vi "get pthread error.vi"(7 "function":T1=enum."pthread_cond_broadcast", 8 "error in (no error)":errorcluster, 11 "errno":i32) -> (0 "error out":errorcluster)   [LabVIEW 2013, in "Linux RT IPC.POSIX Threads.lvlib" / "POSIX Thread Object.lvclass"]
uses:
  <vilib>/NI/NI Linux RT IPC/POSIX Threads/Classes/POSIX Thread Object/POSIX Thread Object.lvclass
  <vilib>/NI/NI Linux RT Errno/Linux Errno.lvlib
  <vilib>/NI/NI Linux RT IPC/POSIX Threads/Classes/POSIX Thread Object/Controls/pthread functions.ctl
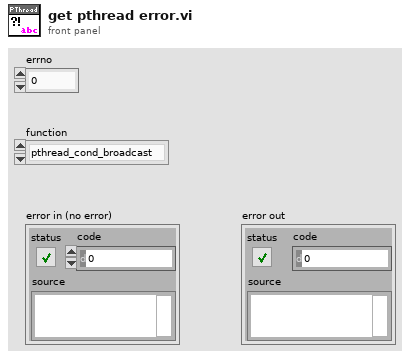
[diagram p1: front panel]
types:
  T1 = typedef "Linux RT IPC.POSIX Threads.lvlib/POSIX Thread Object.lvclass/pthread functions.ctl" = enum16{"unspecified", "pthread_condattr_init", "pthread_condattr_destroy", "pthread_condattr_getclock", "pthread_condattr_setclock", "pthread_condattr_getpshared", "pthread_condattr_setpshared", "pthread_cond_init", "pthread_cond_destroy", "pthread_cond_broadcast", "pthread_cond_signal", "pthread_cond_timedwait", "pthread_cond_wait", "pthread_mutexattr_init", "pthread_mutexattr_destroy", "pthread_mutexattr_getprioceiling", "pthread_mutexattr_setprioceiling", "pthread_mutexattr_getprotocol", "pthread_mutexattr_setprotocol", "pthread_mutexattr_getpshared", "pthread_mutexattr_setpshared", "pthread_mutexattr_gettype", "pthread_mutexattr_settype", "pthread_mutex_init", "pthread_mutex_destroy", "pthread_mutex_getprioceiling", "pthread_mutex_setprioceiling", "pthread_mutex_lock", "pthread_mutex_timedlock", "pthread_mutex_trylock", "pthread_mutex_unlock", "sem_destroy", "sem_getvalue", "sem_init", "sem_open", "sem_post", "sem_timedwait", "sem_trywait", "sem_wait", "barrier_init", "barrier_destroy", "barrier_wait", "barrierattr_init", "barrierattr_destroy", "barrierattr_getpshared", "barrierattr_setpshared"}
  T2 = typedef "Linux Errno.lvlib/errno.ctl" = enum16{"NO ERROR", "EPERM", "ENOENT", "ESRCH", "EINTR", "EIO", "ENXIO", "E2BIG", "ENOEXEC", "EBADF", "ECHILD", "EAGAIN", "ENOMEM", "EACCES", "EFAULT", "ENOTBLK", "EBUSY", "EEXIST", "EXDEV", "ENODEV", "ENOTDIR", "EISDIR", "EINVAL", "ENFILE", "EMFILE", "ENOTTY", "ETXTBSY", "EFBIG", "ENOSPC", "ESPIPE", "EROFS", "EMLINK", "EPIPE", "EDOM", "ERANGE", "EDADLK", "ENAMETOOLONG", "ENOLCK", "ENOSYS", "ENOTEMPTY", "ELOOP", "EWOULDBLOCK", "ENOMSG", "EIDRM", "ECHRNG", "EL2NSYNC", "EL3HLT", "EL3RST", "ELNRNG", "EUNATCH", "ENOCSI", "EL2HLT", "EBADE", "EBADR", "EXFULL", "ENOANO", "EBADRQC", "EBADSLT", "EDEADLOCK", "EBFONT", "ENOSTR", "ENODATA", "ETIME", "ENOSR", "ENONET", "ENOPKG", "EREMOTE", "ENOLINK", "EADV", "ESRMNT", "ECOMM", "EPROTO", "EMULTIHOP", "EDOTDOT", "EBADMSG", "EOVERFLOW", "ENOTUNIQ", "EBADFD", "EREMCHG", "ELIBACC", "ELIBBAD", "ELIBSCN", "ELIBMAX", "ELIBEXEC", "ELISEQ", "ERESTART", "ESTRPIPE", "EUSERS", "ENOTSOCK", "EDESTADDRREQ", "EMSGSIZE", "EPROTOTYPE", "ENOPROTOOPT", "EPROTONOSUPPORT", "ESOCKTNOSUPPORT", "EOPNOTSUPP", "EPFNOSUPPORT", "EAFNOSUPPORT", "EADDRINUSE", "EADDRNOTAVAIL", "ENETDOWN", "ENETUNREACH", "ENETRESET", "ECONNABORTED", "ECONNRESET", "ENOBUFS", "EISCONN", "ENOTCONN", "ESHUTDOWN", "ETOOMANYREFS", "ETIMEDOUT", "ECONNREFUSED", "EHOSTDOWN", "EHOSTUNREACH", "EALREADY", "EINPROGRESS", "ESTALE", "EUCLEAN", "ENOTNAM", "ENAVAIL", "EISNAM", "EREMOTEIO", "EDQUOT", "ENOMEDIUM", "EMEDIUMTYPE", "ECANCELED", "ENOKEY", "EKEYEXPIRED", "EKEYREVOKED", "EKEYREJECTED", "EOWNERDEAD", "ENOTRECOVERABLE", "ERFKILL", "EHWPOISON", "UNDEFINED"}
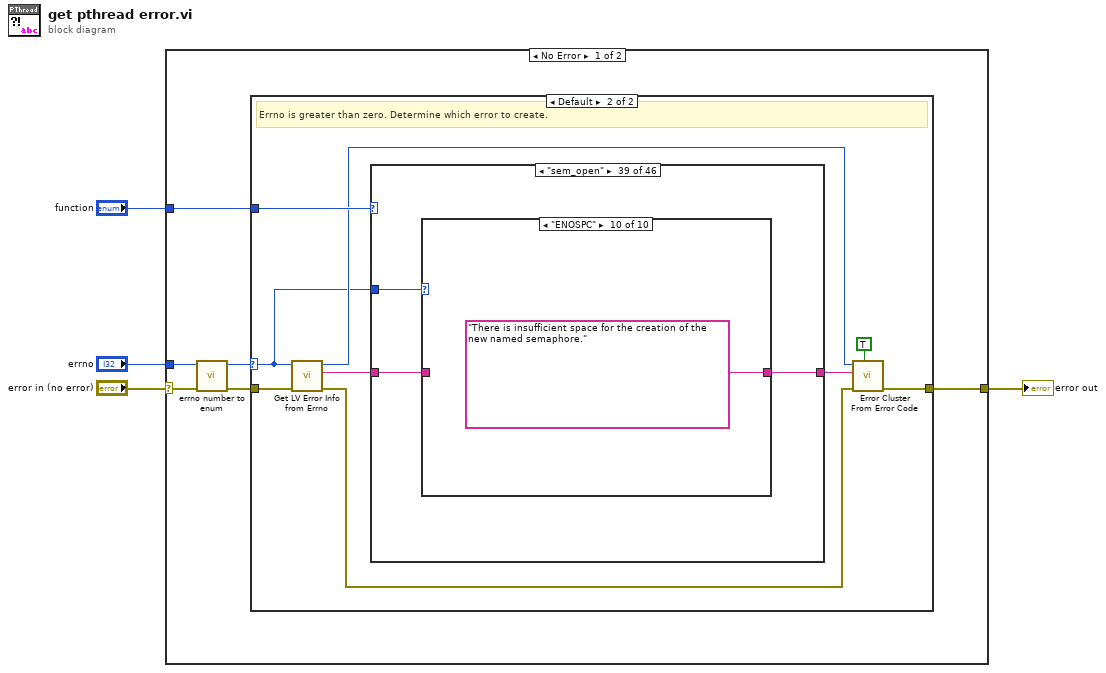
[diagram p0: block diagram]
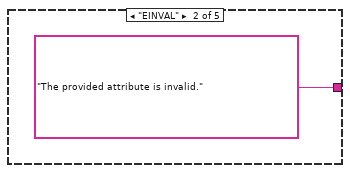
[diagram p5: hidden frame]
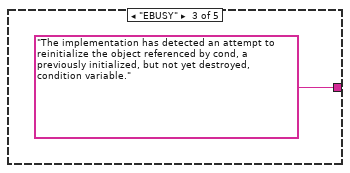
[diagram p6: hidden frame]
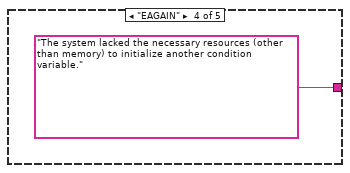
[diagram p7: hidden frame]
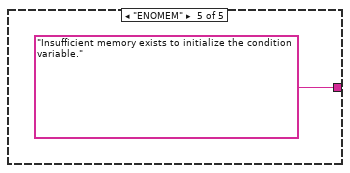
[diagram p8: hidden frame]
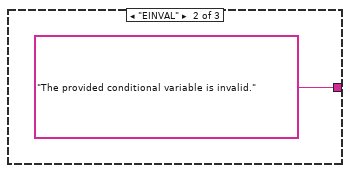
[diagram p10: hidden frame]
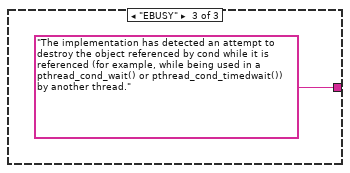
[diagram p11: hidden frame]
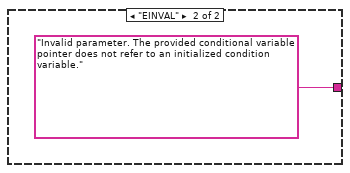
[diagram p13: hidden frame]
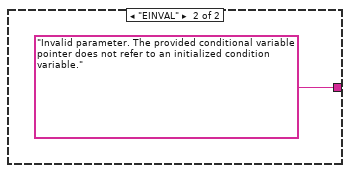
[diagram p15: hidden frame]
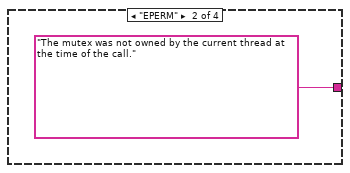
[diagram p17: hidden frame]
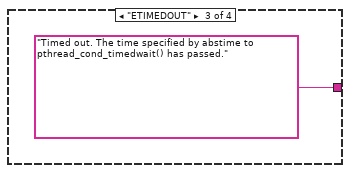
[diagram p18: hidden frame]
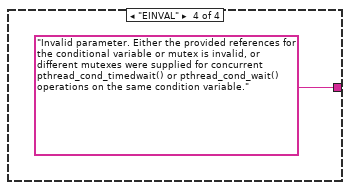
[diagram p19: hidden frame]
diagram:
  n1 = case shown="No Error" "error in (no error)" {
    selector: "error in (no error)" -> [w8 w295]
    tunnel: [w10 w295] -> w3
    tunnel: "errno" -> [w7 _]
    tunnel: "function" -> [w9 _]
    frame No Error {
      n2 = call <vilib>:"errno number to enum.vi"("error in (no error)"=w8, "errno number"=w7) -> ("error out"=w6:errorcluster, "errno enum"=w5:T2)  [unwired: 8 in]
      n3 = case shown="Default" w5 {
        selector: w5 -> [_ w12]
        tunnel: [w11 w20] -> w10
        tunnel: w9 -> [_ w19]
        tunnel: w6 -> [w11 w13]
        frame "NO ERROR" {
          # "Errno is zero. No error occurred."
        }
        frame Default {
          # "Errno is greater than zero. Determine which error to create."
          n4 = call <vilib>:"Get LV Error Info from Errno.vi"("error in (no error)"=w13, "errno"=w12) -> ("error out"=w15:errorcluster, "error description"=w16:string, "error code"=w14:i32)  [unwired: 7 in]
          n5 = case shown="\"sem_open\"" w19 {
            tunnel: w12 -> [_ w24 w32 w38 w43 w48 w55 w61 w66 w71 w76 w81 w86 w91 w96 w101 w107 w113 w119 w126 w131 w136 w141 w146 w155 w161 w167 w173 w181 w189 w196 w203 w208 w213 w219 w225 w232 w239 w245 w258 w266 w272 w277 w282 w287 w292]
            tunnel: [w21 w23 w31 w37 w42 w47 w54 w60 w65 w70 w75 w80 w85 w90 w95 w100 w106 w112 w118 w125 w130 w135 w140 w145 w154 w160 w166 w172 w180 w188 w195 w202 w207 w212 w218 w224 w231 w238 w244 w257 w265 w271 w276 w281 w286 w291] -> w17
            tunnel: w16 -> [w21 w22 w30 w36 w41 w46 w53 w59 w64 w69 w74 w79 w84 w89 w94 w99 w105 w111 w117 w124 w129 w134 w139 w144 w153 w159 w165 w171 w179 w187 w194 w201 w206 w211 w217 w223 w230 w237 w243 w256 w264 w270 w275 w280 w285 w290]
            frame "unspecified", Default {
              # "No specific function was specified, so use generic error description."
            }
            frame "pthread_cond_init" {
              n6 = case shown="\"NO ERROR\", Default" w24 {
                tunnel: [w25 "The provided attribute is invalid." "The implementation has detected an attempt to reinitialize the object referenced by cond, a previously initialized, but not yet destroyed, condition variable." "The system lacked the necessary resources (other than memory) to initialize another condition variable." "Insufficient memory exists to initialize the condition variable."] -> w23
                tunnel: w22 -> [w25 _ _ _ _]
                frame "NO ERROR", Default {
                }
                frame "EINVAL" {
                }
                frame "EBUSY" {
                }
                frame "EAGAIN" {
                }
                frame "ENOMEM" {
                }
              }
            }
            frame "pthread_cond_destroy" {
              n7 = case shown="\"NO ERROR\", Default" w32 {
                tunnel: [w33 "The provided conditional variable is invalid." "The implementation has detected an attempt to destroy the object referenced by cond while it is referenced (for example, while being used in a pthread_cond_wait() or pthread_cond_timedwait()) by another thread."] -> w31
                tunnel: w30 -> [w33 _ _]
                frame "NO ERROR", Default {
                }
                frame "EINVAL" {
                }
                frame "EBUSY" {
                }
              }
            }
            frame "pthread_cond_broadcast" {
              n8 = case shown="\"NO ERROR\", Default" w38 {
                tunnel: [w39 "Invalid parameter. The provided conditional variable pointer does not refer to an initialized condition variable."] -> w37
                tunnel: w36 -> [w39 _]
                frame "NO ERROR", Default {
                }
                frame "EINVAL" {
                }
              }
            }
            frame "pthread_cond_signal" {
              n9 = case shown="\"NO ERROR\", Default" w43 {
                tunnel: [w44 "Invalid parameter. The provided conditional variable pointer does not refer to an initialized condition variable."] -> w42
                tunnel: w41 -> [w44 _]
                frame "NO ERROR", Default {
                }
                frame "EINVAL" {
                }
              }
            }
            frame "pthread_cond_timedwait" {
              n10 = case shown="\"NO ERROR\", Default" w48 {
                tunnel: [w49 "The mutex was not owned by the current thread at the time of the call." "Timed out. The time specified by abstime to pthread_cond_timedwait() has passed." "Invalid parameter. Either the provided references for the conditional variable or mutex is invalid, or different mutexes were supplied for concurrent pthread_cond_timedwait() or pthread_cond_wait() operations on the same condition variable."] -> w47
                tunnel: w46 -> [w49 _ _ _]
                frame "NO ERROR", Default {
                }
                frame "EPERM" {
                }
                frame "ETIMEDOUT" {
                }
                frame "EINVAL" {
                }
              }
            }
            frame "pthread_cond_wait" {
              n11 = case shown="\"NO ERROR\", Default" w55 {
                tunnel: [w56 "The mutex was not owned by the current thread at the time of the call." "Invalid parameter. Either the provided references for the conditional variable or mutex is invalid, or different mutexes were supplied for concurrent pthread_cond_timedwait() or pthread_cond_wait() operations on the same condition variable."] -> w54
                tunnel: w53 -> [w56 _ _]
                frame "NO ERROR", Default {
                }
                frame "EPERM" {
                }
                frame "EINVAL" {
                }
              }
            }
            frame "pthread_condattr_init" {
              n12 = case shown="\"NO ERROR\", Default" w61 {
                tunnel: [w62 "Insufficient memory exists to initialize the condition variable attributes object."] -> w60
                tunnel: w59 -> [w62 _]
                frame "NO ERROR", Default {
                }
                frame "ENOMEM" {
                }
              }
            }
            frame "pthread_condattr_destroy" {
              n13 = case shown="\"NO ERROR\", Default" w66 {
                tunnel: [w67 "The provided condition variable attribute is invalid."] -> w65
                tunnel: w64 -> [w67 _]
                frame "NO ERROR", Default {
                }
                frame "EINVAL" {
                }
              }
            }
            frame "pthread_condattr_getclock" {
              n14 = case shown="\"NO ERROR\", Default" w71 {
                tunnel: [w72 "The provided condition variable attribute is invalid."] -> w70
                tunnel: w69 -> [w72 _]
                frame "NO ERROR", Default {
                }
                frame "EINVAL" {
                }
              }
            }
            frame "pthread_condattr_setclock" {
              n15 = case shown="\"NO ERROR\", Default" w76 {
                tunnel: [w77 "The provided condition variable attribute is invalid, or the value specified by clock_id does not refer to a known clock."] -> w75
                tunnel: w74 -> [w77 _]
                frame "NO ERROR", Default {
                }
                frame "EINVAL" {
                }
              }
            }
            frame "pthread_condattr_getpshared" {
              n16 = case shown="\"NO ERROR\", Default" w81 {
                tunnel: [w82 "The provided condition variable attribute is invalid."] -> w80
                tunnel: w79 -> [w82 _]
                frame "NO ERROR", Default {
                }
                frame "EINVAL" {
                }
              }
            }
            frame "pthread_condattr_setpshared" {
              n17 = case shown="\"NO ERROR\", Default" w86 {
                tunnel: [w87 "The provided condition variable attribute is invalid, or the new value specified for the attribute is outside the range of legal values for that attribute."] -> w85
                tunnel: w84 -> [w87 _]
                frame "NO ERROR", Default {
                }
                frame "EINVAL" {
                }
              }
            }
            frame "pthread_mutexattr_init" {
              n18 = case shown="\"ENOMEM\"" w91 {
                tunnel: [w92 "Insufficient memory exists to initialize the mutex attribute object."] -> w90
                tunnel: w89 -> [w92 _]
                frame "NO ERROR", Default {
                }
                frame "ENOMEM" {
                }
              }
            }
            frame "pthread_mutexattr_destroy" {
              n19 = case shown="\"NO ERROR\", Default" w96 {
                tunnel: [w97 "The value specified by attr is invalid."] -> w95
                tunnel: w94 -> [w97 _]
                frame "NO ERROR", Default {
                }
                frame "EINVAL" {
                }
              }
            }
            frame "pthread_mutexattr_getprioceiling" {
              n20 = case shown="\"NO ERROR\", Default" w101 {
                tunnel: [w102 "The value specified by attr or prioceiling is invalid." "Permission error. The caller does not have the privilege to perform the operation."] -> w100
                tunnel: w99 -> [w102 _ _]
                frame "NO ERROR", Default {
                }
                frame "EINVAL" {
                }
                frame "EPERM" {
                }
              }
            }
            frame "pthread_mutexattr_setprioceiling" {
              n21 = case shown="\"NO ERROR\", Default" w107 {
                tunnel: [w108 "The value specified by attr or prioceiling is invalid." "Permission error. The caller does not have the privilege to perform the operation."] -> w106
                tunnel: w105 -> [w108 _ _]
                frame "NO ERROR", Default {
                }
                frame "EINVAL" {
                }
                frame "EPERM" {
                }
              }
            }
            frame "pthread_mutexattr_getprotocol" {
              n22 = case shown="\"NO ERROR\", Default" w113 {
                tunnel: [w114 "The value specified by attr or protocol is invalid." "The caller does not have the privilege to perform the operation."] -> w112
                tunnel: w111 -> [w114 _ _]
                frame "NO ERROR", Default {
                }
                frame "EINVAL" {
                }
                frame "EPERM" {
                }
              }
            }
            frame "pthread_mutexattr_setprotocol" {
              n23 = case shown="\"NO ERROR\", Default" w119 {
                tunnel: [w120 "The value specified by protocol is an unsupported value." "The value specified by attr or protocol is invalid." "The caller does not have the privilege to perform the operation."] -> w118
                tunnel: w117 -> [w120 _ _ _]
                frame "NO ERROR", Default {
                }
                frame "EOPNOTSUPP" {
                }
                frame "EINVAL" {
                }
                frame "EPERM" {
                }
              }
            }
            frame "pthread_mutexattr_getpshared" {
              n24 = case shown="\"NO ERROR\", Default" w126 {
                tunnel: [w127 "The value specified by attr is invalid."] -> w125
                tunnel: w124 -> [w127 _]
                frame "NO ERROR", Default {
                }
                frame "EINVAL" {
                }
              }
            }
            frame "pthread_mutexattr_setpshared" {
              n25 = case shown="\"NO ERROR\", Default" w131 {
                tunnel: [w132 "The value specified by attr is invalid, or the new value specified for the attribute is outside the range of legal values for that attribute."] -> w130
                tunnel: w129 -> [w132 _]
                frame "NO ERROR", Default {
                }
                frame "EINVAL" {
                }
              }
            }
            frame "pthread_mutexattr_gettype" {
              n26 = case shown="\"NO ERROR\", Default" w136 {
                tunnel: [w137 "The value specified by attr is invalid."] -> w135
                tunnel: w134 -> [w137 _]
                frame "NO ERROR", Default {
                }
                frame "EINVAL" {
                }
              }
            }
            frame "pthread_mutexattr_settype" {
              n27 = case shown="\"NO ERROR\", Default" w141 {
                tunnel: [w142 "The value specified by attr is invalid, or the value type is invalid."] -> w140
                tunnel: w139 -> [w142 _]
                frame "NO ERROR", Default {
                }
                frame "EINVAL" {
                }
              }
            }
            frame "pthread_mutex_init" {
              n28 = case shown="\"NO ERROR\", Default" w146 {
                tunnel: [w147 "The provided mutex attribute is invalid." "The implementation has detected an attempt to  reinitialize the object referenced by mutex, a previously initialized, but not yet destroyed, mutex." "Permission error. The caller does not have the privilege to perform the operation." "Insufficient memory exists to initialize the mutex." "The system lacked the necessary resources (other than memory) to initialize another mutex."] -> w145
                tunnel: w144 -> [w147 _ _ _ _ _]
                frame "NO ERROR", Default {
                }
                frame "EINVAL" {
                }
                frame "EBUSY" {
                }
                frame "EPERM" {
                }
                frame "ENOMEM" {
                }
                frame "EAGAIN" {
                }
              }
            }
            frame "pthread_mutex_destroy" {
              n29 = case shown="\"NO ERROR\", Default" w155 {
                tunnel: [w156 "The provided mutex is invalid." "The implementation has detected an attempt to destroy the object referenced by mutex while it is locked or referenced (for  example, while being used in a pthread_cond_timedwait() or pthread_cond_wait()) by another thread."] -> w154
                tunnel: w153 -> [w156 _ _]
                frame "NO ERROR", Default {
                }
                frame "EINVAL" {
                }
                frame "EBUSY" {
                }
              }
            }
            frame "pthread_mutex_getprioceiling" {
              n30 = case shown="\"NO ERROR\", Default" w161 {
                tunnel: [w162 "The value specified by mutex does not refer to a currently existing mutex." "Permission error. The caller does not have the privilege to perform the operation."] -> w160
                tunnel: w159 -> [w162 _ _]
                frame "NO ERROR", Default {
                }
                frame "EINVAL" {
                }
                frame "EPERM" {
                }
              }
            }
            frame "pthread_mutex_setprioceiling" {
              n31 = case shown="\"NO ERROR\", Default" w167 {
                tunnel: [w168 "The value specified by mutex does not refer to a currently existing mutex, or the priority requested by priority ceiling is out of range." "Permission error. The caller does not have the privilege to perform the operation."] -> w166
                tunnel: w165 -> [w168 _ _]
                frame "NO ERROR", Default {
                }
                frame "EINVAL" {
                }
                frame "EPERM" {
                }
              }
            }
            frame "pthread_mutex_lock" {
              n32 = case shown="\"NO ERROR\", Default" w173 {
                tunnel: [w174 "Invalid parameter. Either the provided mutex reference does not refer to an initialized mutex object, or the mutex was created with the protocol attribute having the value PTHREAD_PRIO_PROTECT and the calling thread's priority is higher than the mutex's current priority ceiling." "The mutex could not be acquired because the maximum number of recursive locks for mutex has been exceeded." "Deadlock avoided. The current thread already owns the mutex." "Deadlock avoided. The current thread already owns the mutex."] -> w172
                tunnel: w171 -> [w174 _ _ _ _]
                frame "NO ERROR", Default {
                }
                frame "EINVAL" {
                }
                frame "EAGAIN" {
                }
                frame "EDEADLOCK" {
                }
                frame "EDADLK" {
                }
              }
            }
            frame "pthread_mutex_timedlock" {
              n33 = case shown="\"NO ERROR\", Default" w181 {
                tunnel: [w182 "Invalid parameter. One of the following parameters was invalid:\n\nThe value specified by mutex does not refer to an initialized mutex object.\n\nThe mutex was created with the protocol attribute having the value PTHREAD_PRIO_PROTECT and the calling thread's priority is higher than the mutex's current priority ceiling." "The mutex could not be locked before the specified timeout expired." "The mutex could not be acquired because the maximum number of recursive locks for mutex has been exceeded." "The current thread already owns the mutex."] -> w180
                tunnel: w179 -> [w182 _ _ _ _]
                frame "NO ERROR", Default {
                }
                frame "EINVAL" {
                }
                frame "ETIMEDOUT" {
                }
                frame "EAGAIN" {
                }
                frame "EDEADLOCK" {
                }
              }
            }
            frame "pthread_mutex_trylock" {
              n34 = case shown="\"NO ERROR\", Default" w189 {
                tunnel: [w190 "Invalid parameter. Either the provided mutex reference does not refer to an initialized mutex object, or the mutex was created with the protocol attribute having the value PTHREAD_PRIO_PROTECT and the calling thread's priority is higher than the mutex's current priority ceiling." "The mutex could not be acquired because the maximum number of recursive locks for mutex has been exceeded." "The mutex could not be acquired because it was already locked."] -> w188
                tunnel: w187 -> [w190 _ _ _]
                frame "NO ERROR", Default {
                }
                frame "EINVAL" {
                }
                frame "EAGAIN" {
                }
                frame "EBUSY" {
                }
              }
            }
            frame "pthread_mutex_unlock" {
              n35 = case shown="\"NO ERROR\", Default" w196 {
                tunnel: [w197 "Invalid parameter. The provided mutex reference does not refer to an initialized mutex object." "The mutex could not be acquired because the maximum number of recursive locks for mutex has been exceeded." "The current thread does not own the mutex."] -> w195
                tunnel: w194 -> [w197 _ _ _]
                frame "NO ERROR", Default {
                }
                frame "EINVAL" {
                }
                frame "EAGAIN" {
                }
                frame "EPERM" {
                }
              }
            }
            frame "sem_destroy" {
              n36 = case shown="\"NO ERROR\", Default" w203 {
                tunnel: [w204 "sem is not a valid semaphore."] -> w202
                tunnel: w201 -> [w204 _]
                frame "NO ERROR", Default {
                }
                frame "EINVAL" {
                }
              }
            }
            frame "sem_getvalue" {
              n37 = case shown="\"EINVAL\"" w208 {
                tunnel: [w209 "sem is not a valid semaphore."] -> w207
                tunnel: w206 -> [w209 _]
                frame "NO ERROR", Default {
                }
                frame "EINVAL" {
                }
              }
            }
            frame "sem_init" {
              n38 = case shown="\"ENOSYS\"" w213 {
                tunnel: [w214 "Value exceeds SEM_VALUE_MAX." "Semaphore is set to be shared, but the system does not support process-shared semaphores."] -> w212
                tunnel: w211 -> [w214 _ _]
                frame "NO ERROR", Default {
                }
                frame "EINVAL" {
                }
                frame "ENOSYS" {
                }
              }
            }
            frame "sem_post" {
              n39 = case shown="\"EOVERFLOW\"" w219 {
                tunnel: [w220 "sem is not a valid semaphore." "The maximum allowable value for a semaphore would be exceeded."] -> w218
                tunnel: w217 -> [w220 _ _]
                frame "NO ERROR", Default {
                }
                frame "EINVAL" {
                }
                frame "EOVERFLOW" {
                }
              }
            }
            frame "sem_timedwait" {
              n40 = case shown="\"NO ERROR\", Default" w225 {
                tunnel: [w226 "Either sem is not a valid semaphore, or the nanosecond value of the provided timespec is less than 0, or greater than or equal to 1 billion." "The call was interrupted by a signal handler." "The call timed out before the semaphore could be locked."] -> w224
                tunnel: w223 -> [w226 _ _ _]
                frame "NO ERROR", Default {
                }
                frame "EINVAL" {
                }
                frame "EINTR" {
                }
                frame "ETIMEDOUT" {
                }
              }
            }
            frame "sem_trywait" {
              n41 = case shown="\"EAGAIN\"" w232 {
                tunnel: [w233 "sem is not a valid semaphore." "The call was interrupted by a signal handler." "The operation could not be performed without blocking (i.e., the semaphore currently has the value zero)."] -> w231
                tunnel: w230 -> [w233 _ _ _]
                frame "NO ERROR", Default {
                }
                frame "EINVAL" {
                }
                frame "EINTR" {
                }
                frame "EAGAIN" {
                }
              }
            }
            frame "sem_wait" {
              n42 = case shown="\"EINVAL\"" w239 {
                tunnel: [w240 "sem is not a valid semaphore." "The call was interrupted by a signal handler."] -> w238
                tunnel: w237 -> [w240 _ _]
                frame "NO ERROR", Default {
                }
                frame "EINVAL" {
                }
                frame "EINTR" {
                }
              }
            }
            frame "sem_open" {
              n43 = case shown="\"ENOSPC\"" w245 {
                tunnel: [w246 "The sem_open() operation is not supported for the given name, or O_CREAT was specified in oflag and value was greater than {SEM_VALUE_MAX}." "The named semaphore exists and the permissions specified by oflag are denied, or the named semaphore does not exist and permission to create the named semaphore is denied." "O_CREAT and O_EXCL are set and the named semaphore already exists." "The sem_open() operation was interrupted by a signal." "Too many semaphore descriptors or file descriptors are currently in use by this process." "The length of the name argument exceeds {PATH_MAX} or a pathname component is longer than {NAME_MAX}." "Too many semaphores are currently open in the system." "O_CREAT is not set and the named semaphore does not exist." "There is insufficient space for the creation of the new named semaphore."] -> w244
                tunnel: w243 -> [w246 _ _ _ _ _ _ _ _ _]
                frame "NO ERROR", Default {
                }
                frame "EINVAL" {
                }
                frame "EACCES" {
                }
                frame "EEXIST" {
                }
                frame "EINTR" {
                }
                frame "EMFILE" {
                }
                frame "ENAMETOOLONG" {
                }
                frame "ENFILE" {
                }
                frame "ENOENT" {
                }
                frame "ENOSPC" {
                }
              }
            }
            frame "barrier_init" {
              n44 = case shown="\"NO ERROR\", Default" w258 {
                tunnel: [w259 "Invalid argument. The provided barrier attribute object is not valid, or the provided count is not valid." "The implementation has detected an attempt to reinitialize a barrier while it is in use (for example, while being used in a pthread_barrier_wait() call) by another thread." "The system lacks the necessary resources to initialize another barrier." "Insufficient memory exists to initialize the barrier."] -> w257
                tunnel: w256 -> [w259 _ _ _ _]
                frame "NO ERROR", Default {
                }
                frame "EINVAL" {
                }
                frame "EBUSY" {
                }
                frame "EAGAIN" {
                }
                frame "ENOMEM" {
                }
              }
            }
            frame "barrier_destroy" {
              n45 = case shown="\"EBUSY\"" w266 {
                tunnel: [w267 "Invalid argument. The provided barrier is invalid." "The implementation has detected an attempt to destroy a barrier while it is in use (for example, while being used in a pthread_barrier_wait() call) by another thread."] -> w265
                tunnel: w264 -> [w267 _ _]
                frame "NO ERROR", Default {
                }
                frame "EINVAL" {
                }
                frame "EBUSY" {
                }
              }
            }
            frame "barrier_wait" {
              n46 = case shown="\"EINVAL\"" w272 {
                tunnel: [w273 "The value specified by barrier does not refer to an initialized barrier object."] -> w271
                tunnel: w270 -> [w273 _]
                frame "NO ERROR", Default {
                }
                frame "EINVAL" {
                }
              }
            }
            frame "barrierattr_init" {
              n47 = case shown="\"ENOMEM\"" w277 {
                tunnel: [w278 "Insufficient memory exists to initialize the barrier attributes object."] -> w276
                tunnel: w275 -> [w278 _]
                frame "NO ERROR", Default {
                }
                frame "ENOMEM" {
                }
              }
            }
            frame "barrierattr_destroy" {
              n48 = case shown="\"EINVAL\"" w282 {
                tunnel: [w283 "The value specified by barrier attr is invalid."] -> w281
                tunnel: w280 -> [w283 _]
                frame "NO ERROR", Default {
                }
                frame "EINVAL" {
                }
              }
            }
            frame "barrierattr_getpshared" {
              n49 = case shown="\"EINVAL\"" w287 {
                tunnel: [w288 "The value specified by barrier attr is invalid."] -> w286
                tunnel: w285 -> [w288 _]
                frame "NO ERROR", Default {
                }
                frame "EINVAL" {
                }
              }
            }
            frame "barrierattr_setpshared" {
              n50 = case shown="\"EINVAL\"" w292 {
                tunnel: [w293 "The value specified by barrier attr is invalid, or the provided value for the process-shared attribute is no the value of PTHREAD_PROCESS_SHARED or PTHREAD_PROCESS_PRIVATE."] -> w291
                tunnel: w290 -> [w293 _]
                frame "NO ERROR", Default {
                }
                frame "EINVAL" {
                }
              }
            }
          }
          n51 = call <vilib>:"Error Cluster From Error Code.vi"("show call chain? (False)"=TRUE, "error in (no error)"=w15, "error message (\"\")"=w17, "error code (0)"=w14) -> ("error out"=w20:errorcluster)  [unwired: 5 in]
        }
      }
    }
    frame Error {
      # "Error already exists. Pass through."
    }
  }
  "error out" <- w3
